vi "Test Log.vi"() -> ()   [LabVIEW 2018, in "System Log.lvclass"]
uses:
  System Log.lvclass
  <vilib>/MSR Consulting, LLC/General Reuse/Session APIs/_Session Fwk/Session - Root.lvclass
  C:/Program Files (x86)/National Instruments/LabVIEW 2018/vi.lib/MSR Consulting, LLC/General Reuse/Session APIs/_Session Fwk/Session - Root.lvclass
panel:
  in  "showFP":bool
  out "error out":errorcluster
  in  "logevent":bool
  in  "Msg":string
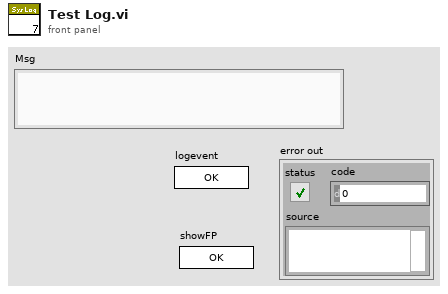
[diagram p1: front panel]
types:
  T1 = typedef "Session - Root.lvclass/Session Handle.ctl" = refnum<data-value>
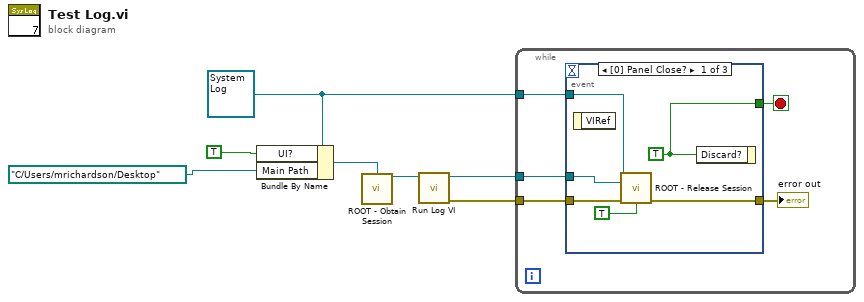
[diagram p0: block diagram]
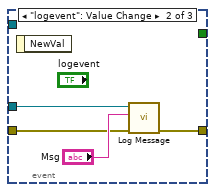
[diagram p2: hidden frame]
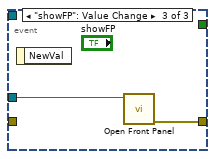
[diagram p3: hidden frame]
diagram:
  w4 = refnum<class "System Log.lvclass"> refnum ("Sys Log")
  n1 = Bundle By Name(cluster=w4, "UI?"=TRUE, "Main Path"=path "C:/Users/mrichardson/Desktop") -> (w5:refnum<class "System Log.lvclass">)
  n2 = call <vilib>:"ROOT - Obtain Session.vi"("OBJ - Session"=w5) -> ("Session Handle"=w3:T1)  [unwired: 12 in, 2 out]
  n3 = call "Run Log VI.vi"("Session Handle In"=w3) -> ("error out"=w1:errorcluster, "Session Handle Out"=w2:T1)  [unwired: 9 in]
  n4 = while {
    tunnel: w2 -> [w11]
    tunnel: w4 -> [w10]
    tunnel: w1 -> [w8]
    stop <- w12 stop-if-true
    n5 = event shown="[0] Panel Close?" {
      selector: _ -> [_ _ _]
      dyn-events: _ -> [_ _ _]
      timeout: _ -> [_ _ _]
      tunnel: [w18 _ _] -> w12
      tunnel: w11 -> [w17 w20 w24]
      tunnel: w10 -> [w16 _ _]
      tunnel: [w15 w21 w23] -> w9
      tunnel: w8 -> [w13 w19 _]
      event Panel Close? {
        w18 = TRUE ("Discard?")
        n6 = event-data() -> ()  [unwired: 1 in, 1 out]
        n7 = call <vilib>:"ROOT - Release Session.vi"("OBJ - Session in"=w16, "Session Handle in"=w17, "error in (no error)"=w13, "force destroy? (F)"=TRUE) -> ("error out"=w15:errorcluster)  [unwired: 10 in, 1 out]
        n8 = event-data("Discard?"=w18) -> ()  [unwired: 1 in, 1 out]
      }
      event "logevent": Value Change {
        n9 = event-data() -> ()  [unwired: 1 in, 1 out]
        n10 = call "Log Message.vi"("error in"=w19, "MSG In"="Msg", "session in"=w20) -> ("error out"=w21:errorcluster)  [unwired: 7 in, 1 out]
      }
      event "showFP": Value Change {
        n11 = event-data() -> ()  [unwired: 1 in, 1 out]
        n12 = call "Open Front Panel.vi"("Session In"=w24) -> ("error out"=w23:errorcluster)  [unwired: 9 in, 1 out]
      }
    }
    "error out" <- w9
  }
